vi "Status Created Events.vi"(11 "qqqqq in":refnum<class "qqqqq.lvclass">) -> (0 "Created Event Count":i32, 1 "Created Event Aliases":string[](array[string]), 2 "Created Event Exist?":bool, 3 "qqqqq out":refnum<class "qqqqq.lvclass">)   [LabVIEW 2021, in "jettl Tools.lvlib" / "qqqqq.lvlib" / "qqqqq.lvclass"]
uses:
  qqqqq.lvclass
  qqqqq.lvclass/qqqqq.ctl
  jettl/Queue/Queue.lvclass
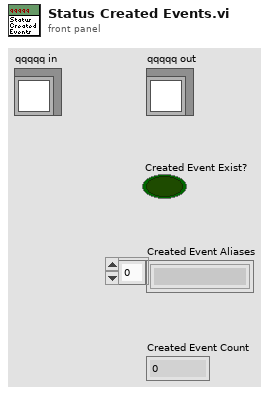
[diagram p1: front panel]
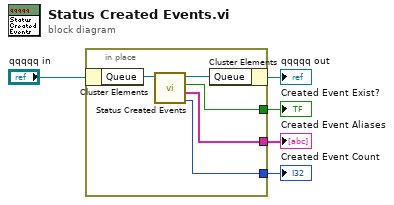
[diagram p0: block diagram]
diagram:
  n1 = in-place {
    in-place-border: [w8] -> w3
    in-place-border: [w7] -> w2
    in-place-border: [w6] -> w1
    n2 = in-place-cluster #1("qqqqq in") -> ("Queue"=w10:refnum<class "Queue.lvclass">)
    n3 = call-dynamic "Status Created Events.vi"("Queue in"=w10) -> ("Created Event Count"=w6:i32, "Created Event Aliases"=w7:string[], "Created Event Exist?"=w8:bool, "Queue out"=w9:refnum<class "Queue.lvclass">)  [unwired: 7 in]
    n4 = in-place-cluster #1("Queue"=w9) -> (→"qqqqq out":refnum<class "qqqqq.lvclass">)
  }
  "Created Event Aliases" <- w2
  "Created Event Count" <- w1
  "Created Event Exist?" <- w3
